vi "WellPartition_Index.vi"(2 "PartitionArray":string[](array[string])=["A, MQ unfiltered", "A, MQ unfiltered", "A, MQ unfiltered", "B, D2O unfiltered", "B, D2O unfiltered", "B, D2O unfiltered", "C, 1mg/ml Snomax in MQ", "C, 1mg/ml Snomax in MQ", "C, 1mg/ml Snomax in MQ", "C, 1mg/ml Snomax in MQ", "C, 1mg/ml Snomax in MQ", "C, 1mg/ml Snomax in MQ", "D, 1mg/ml Snomax in 1:1 MQ:D2O", "D, 1mg/ml Snomax in 1:1 MQ:D2O", "D, 1mg/ml Snomax in 1:1 MQ:D2O", "D, 1mg/ml Snomax in 1:1 MQ:D2O", "D, 1mg/ml Snomax in 1:1 MQ:D2O", "D, 1mg/ml Snomax in 1:1 MQ:D2O", "E, 1mg/ml Snomax in D2O", "E, 1mg/ml Snomax in D2O", "E, 1mg/ml Snomax in D2O", "E, 1mg/ml Snomax in D2O", "E, 1mg/ml Snomax in D2O", "E, 1mg/ml Snomax in D2O", "A, MQ unfiltered", "A, MQ unfiltered", "A, MQ unfiltered", "B, D2O unfiltered", "B, D2O unfiltered", "B, D2O unfiltered", "C, 1mg/ml Snomax in MQ", "C, 1mg/ml Snomax in MQ", "C, 1mg/ml Snomax in MQ", "C, 1mg/ml Snomax in MQ", "C, 1mg/ml Snomax in MQ", "C, 1mg/ml Snomax in MQ", "D, 1mg/ml Snomax in 1:1 MQ:D2O", "D, 1mg/ml Snomax in 1:1 MQ:D2O", "D, 1mg/ml Snomax in 1:1 MQ:D2O", "D, 1mg/ml Snomax in 1:1 MQ:D2O", "D, 1mg/ml Snomax in 1:1 MQ:D2O", "D, 1mg/ml Snomax in 1:1 MQ:D2O", "E, 1mg/ml Snomax in D2O", "E, 1mg/ml Snomax in D2O", "E, 1mg/ml Snomax in D2O", "E, 1mg/ml Snomax in D2O", "E, 1mg/ml Snomax in D2O", "E, 1mg/ml Snomax in D2O", "A, MQ unfiltered", "A, MQ unfiltered", "A, MQ unfiltered", "B, D2O unfiltered", "B, D2O unfiltered", "B, D2O unfiltered", "C, 1mg/ml Snomax in MQ", "C, 1mg/ml Snomax in MQ", "C, 1mg/ml Snomax in MQ", "C, 1mg/ml Snomax in MQ", "C, 1mg/ml Snomax in MQ", "C, 1mg/ml Snomax in MQ", "D, 1mg/ml Snomax in 1:1 MQ:D2O", "D, 1mg/ml Snomax in 1:1 MQ:D2O", "D, 1mg/ml Snomax in 1:1 MQ:D2O", "D, 1mg/ml Snomax in 1:1 MQ:D2O", "D, 1mg/ml Snomax in 1:1 MQ:D2O", "D, 1mg/ml Snomax in 1:1 MQ:D2O", "E, 1mg/ml Snomax in D2O", "E, 1mg/ml Snomax in D2O", "E, 1mg/ml Snomax in D2O", "E, 1mg/ml Snomax in D2O", "E, 1mg/ml Snomax in D2O", "E, 1mg/ml Snomax in D2O", "A, MQ unfiltered", "A, MQ unfiltered", "A, MQ unfiltered", "B, D2O unfiltered", "B, D2O unfiltered", "B, D2O unfiltered", "C, 1mg/ml Snomax in MQ", "C, 1mg/ml Snomax in MQ", "C, 1mg/ml Snomax in MQ", "C, 1mg/ml Snomax in MQ", "C, 1mg/ml Snomax in MQ", "C, 1mg/ml Snomax in MQ", "D, 1mg/ml Snomax in 1:1 MQ:D2O", "D, 1mg/ml Snomax in 1:1 MQ:D2O", "D, 1mg/ml Snomax in 1:1 MQ:D2O", "D, 1mg/ml Snomax in 1:1 MQ:D2O", "D, 1mg/ml Snomax in 1:1 MQ:D2O", "D, 1mg/ml Snomax in 1:1 MQ:D2O", "E, 1mg/ml Snomax in D2O", "E, 1mg/ml Snomax in D2O", "E, 1mg/ml Snomax in D2O", "E, 1mg/ml Snomax in D2O", "E, 1mg/ml Snomax in D2O", "E, 1mg/ml Snomax in D2O", "A, MQ unfiltered", "A, MQ unfiltered", "A, MQ unfiltered", "B, D2O unfiltered", "B, D2O unfiltered", "B, D2O unfiltered", "C, 1mg/ml Snomax in MQ", "C, 1mg/ml Snomax in MQ", "C, 1mg/ml Snomax in MQ", "C, 1mg/ml Snomax in MQ", "C, 1mg/ml Snomax in MQ", "C, 1mg/ml Snomax in MQ", "D, 1mg/ml Snomax in 1:1 MQ:D2O", "D, 1mg/ml Snomax in 1:1 MQ:D2O", "D, 1mg/ml Snomax in 1:1 MQ:D2O", "D, 1mg/ml Snomax in 1:1 MQ:D2O", "D, 1mg/ml Snomax in 1:1 MQ:D2O", "D, 1mg/ml Snomax in 1:1 MQ:D2O", "E, 1mg/ml Snomax in D2O", "E, 1mg/ml Snomax in D2O", "E, 1mg/ml Snomax in D2O", "E, 1mg/ml Snomax in D2O", "E, 1mg/ml Snomax in D2O", "E, 1mg/ml Snomax in D2O", "A, MQ unfiltered", "A, MQ unfiltered", "A, MQ unfiltered", "B, D2O unfiltered", "B, D2O unfiltered", "B, D2O unfiltered", "C, 1mg/ml Snomax in MQ", "C, 1mg/ml Snomax in MQ", "C, 1mg/ml Snomax in MQ", "C, 1mg/ml Snomax in MQ", "C, 1mg/ml Snomax in MQ", "C, 1mg/ml Snomax in MQ", "D, 1mg/ml Snomax in 1:1 MQ:D2O", "D, 1mg/ml Snomax in 1:1 MQ:D2O", "D, 1mg/ml Snomax in 1:1 MQ:D2O", "D, 1mg/ml Snomax in 1:1 MQ:D2O", "D, 1mg/ml Snomax in 1:1 MQ:D2O", "D, 1mg/ml Snomax in 1:1 MQ:D2O", "E, 1mg/ml Snomax in D2O", "E, 1mg/ml Snomax in D2O", "E, 1mg/ml Snomax in D2O", "E, 1mg/ml Snomax in D2O", "E, 1mg/ml Snomax in D2O", "E, 1mg/ml Snomax in D2O", "A, MQ unfiltered", "A, MQ unfiltered", "A, MQ unfiltered", "B, D2O unfiltered", "B, D2O unfiltered", "B, D2O unfiltered", "C, 1mg/ml Snomax in MQ", "C, 1mg/ml Snomax in MQ", "C, 1mg/ml Snomax in MQ", "C, 1mg/ml Snomax in MQ", "C, 1mg/ml Snomax in MQ", "C, 1mg/ml Snomax in MQ", "D, 1mg/ml Snomax in 1:1 MQ:D2O", "D, 1mg/ml Snomax in 1:1 MQ:D2O", "D, 1mg/ml Snomax in 1:1 MQ:D2O", "D, 1mg/ml Snomax in 1:1 MQ:D2O", "D, 1mg/ml Snomax in 1:1 MQ:D2O", "D, 1mg/ml Snomax in 1:1 MQ:D2O", "E, 1mg/ml Snomax in D2O", "E, 1mg/ml Snomax in D2O", "E, 1mg/ml Snomax in D2O", "E, 1mg/ml Snomax in D2O", "E, 1mg/ml Snomax in D2O", "E, 1mg/ml Snomax in D2O", "A, MQ unfiltered", "A, MQ unfiltered", "A, MQ unfiltered", "B, D2O unfiltered", "B, D2O unfiltered", "B, D2O unfiltered", "C, 1mg/ml Snomax in MQ", "C, 1mg/ml Snomax in MQ", "C, 1mg/ml Snomax in MQ", "C, 1mg/ml Snomax in MQ", "C, 1mg/ml Snomax in MQ", "C, 1mg/ml Snomax in MQ", "D, 1mg/ml Snomax in 1:1 MQ:D2O", "D, 1mg/ml Snomax in 1:1 MQ:D2O", "D, 1mg/ml Snomax in 1:1 MQ:D2O", "D, 1mg/ml Snomax in 1:1 MQ:D2O", "D, 1mg/ml Snomax in 1:1 MQ:D2O", "D, 1mg/ml Snomax in 1:1 MQ:D2O", "E, 1mg/ml Snomax in D2O", "E, 1mg/ml Snomax in D2O", "E, 1mg/ml Snomax in D2O", "E, 1mg/ml Snomax in D2O", "E, 1mg/ml Snomax in D2O", "E, 1mg/ml Snomax in D2O", "A, MQ unfiltered", "A, MQ unfiltered", "A, MQ unfiltered", "B, D2O unfiltered", "B, D2O unfiltered", "B, D2O unfiltered", "C, 1mg/ml Snomax in MQ", "C, 1mg/ml Snomax in MQ", "C, 1mg/ml Snomax in MQ", "C, 1mg/ml Snomax in MQ", "C, 1mg/ml Snomax in MQ", "C, 1mg/ml Snomax in MQ", "D, 1mg/ml Snomax in 1:1 MQ:D2O", "D, 1mg/ml Snomax in 1:1 MQ:D2O", "D, 1mg/ml Snomax in 1:1 MQ:D2O", "D, 1mg/ml Snomax in 1:1 MQ:D2O", "D, 1mg/ml Snomax in 1:1 MQ:D2O", "D, 1mg/ml Snomax in 1:1 MQ:D2O", "E, 1mg/ml Snomax in D2O", "E, 1mg/ml Snomax in D2O", "E, 1mg/ml Snomax in D2O", "E, 1mg/ml Snomax in D2O", "E, 1mg/ml Snomax in D2O", "E, 1mg/ml Snomax in D2O", "A, MQ unfiltered", "A, MQ unfiltered", "A, MQ unfiltered", "B, D2O unfiltered", "B, D2O unfiltered", "B, D2O unfiltered", "C, 1mg/ml Snomax in MQ", "C, 1mg/ml Snomax in MQ", "C, 1mg/ml Snomax in MQ", "C, 1mg/ml Snomax in MQ", "C, 1mg/ml Snomax in MQ", "C, 1mg/ml Snomax in MQ", "D, 1mg/ml Snomax in 1:1 MQ:D2O", "D, 1mg/ml Snomax in 1:1 MQ:D2O", "D, 1mg/ml Snomax in 1:1 MQ:D2O", "D, 1mg/ml Snomax in 1:1 MQ:D2O", "D, 1mg/ml Snomax in 1:1 MQ:D2O", "D, 1mg/ml Snomax in 1:1 MQ:D2O", "E, 1mg/ml Snomax in D2O", "E, 1mg/ml Snomax in D2O", "E, 1mg/ml Snomax in D2O", "E, 1mg/ml Snomax in D2O", "E, 1mg/ml Snomax in D2O", "E, 1mg/ml Snomax in D2O", "A, MQ unfiltered", "A, MQ unfiltered", "A, MQ unfiltered", "B, D2O unfiltered", "B, D2O unfiltered", "B, D2O unfiltered", "C, 1mg/ml Snomax in MQ", "C, 1mg/ml Snomax in MQ", "C, 1mg/ml Snomax in MQ", "C, 1mg/ml Snomax in MQ", "C, 1mg/ml Snomax in MQ", "C, 1mg/ml Snomax in MQ", "D, 1mg/ml Snomax in 1:1 MQ:D2O", "D, 1mg/ml Snomax in 1:1 MQ:D2O", "D, 1mg/ml Snomax in 1:1 MQ:D2O", "D, 1mg/ml Snomax in 1:1 MQ:D2O", "D, 1mg/ml Snomax in 1:1 MQ:D2O", "D, 1mg/ml Snomax in 1:1 MQ:D2O", "E, 1mg/ml Snomax in D2O", "E, 1mg/ml Snomax in D2O", "E, 1mg/ml Snomax in D2O", "E, 1mg/ml Snomax in D2O", "E, 1mg/ml Snomax in D2O", "E, 1mg/ml Snomax in D2O", "A, MQ unfiltered", "A, MQ unfiltered", "A, MQ unfiltered", "B, D2O unfiltered", "B, D2O unfiltered", "B, D2O unfiltered", "C, 1mg/ml Snomax in MQ", "C, 1mg/ml Snomax in MQ", "C, 1mg/ml Snomax in MQ", "C, 1mg/ml Snomax in MQ", "C, 1mg/ml Snomax in MQ", "C, 1mg/ml Snomax in MQ", "D, 1mg/ml Snomax in 1:1 MQ:D2O", "D, 1mg/ml Snomax in 1:1 MQ:D2O", "D, 1mg/ml Snomax in 1:1 MQ:D2O", "D, 1mg/ml Snomax in 1:1 MQ:D2O", "D, 1mg/ml Snomax in 1:1 MQ:D2O", "D, 1mg/ml Snomax in 1:1 MQ:D2O", "E, 1mg/ml Snomax in D2O", "E, 1mg/ml Snomax in D2O", "E, 1mg/ml Snomax in D2O", "E, 1mg/ml Snomax in D2O", "E, 1mg/ml Snomax in D2O", "E, 1mg/ml Snomax in D2O", "A, MQ unfiltered", "A, MQ unfiltered", "A, MQ unfiltered", "B, D2O unfiltered", "B, D2O unfiltered", "B, D2O unfiltered", "C, 1mg/ml Snomax in MQ", "C, 1mg/ml Snomax in MQ", "C, 1mg/ml Snomax in MQ", "C, 1mg/ml Snomax in MQ", "C, 1mg/ml Snomax in MQ", "C, 1mg/ml Snomax in MQ", "D, 1mg/ml Snomax in 1:1 MQ:D2O", "D, 1mg/ml Snomax in 1:1 MQ:D2O", "D, 1mg/ml Snomax in 1:1 MQ:D2O", "D, 1mg/ml Snomax in 1:1 MQ:D2O", "D, 1mg/ml Snomax in 1:1 MQ:D2O", "D, 1mg/ml Snomax in 1:1 MQ:D2O", "E, 1mg/ml Snomax in D2O", "E, 1mg/ml Snomax in D2O", "E, 1mg/ml Snomax in D2O", "E, 1mg/ml Snomax in D2O", "E, 1mg/ml Snomax in D2O", "E, 1mg/ml Snomax in D2O", "A, MQ unfiltered", "A, MQ unfiltered", "A, MQ unfiltered", "B, D2O unfiltered", "B, D2O unfiltered", "B, D2O unfiltered", "C, 1mg/ml Snomax in MQ", "C, 1mg/ml Snomax in MQ", "C, 1mg/ml Snomax in MQ", "C, 1mg/ml Snomax in MQ", "C, 1mg/ml Snomax in MQ", "C, 1mg/ml Snomax in MQ", "D, 1mg/ml Snomax in 1:1 MQ:D2O", "D, 1mg/ml Snomax in 1:1 MQ:D2O", "D, 1mg/ml Snomax in 1:1 MQ:D2O", "D, 1mg/ml Snomax in 1:1 MQ:D2O", "D, 1mg/ml Snomax in 1:1 MQ:D2O", "D, 1mg/ml Snomax in 1:1 MQ:D2O", "E, 1mg/ml Snomax in D2O", "E, 1mg/ml Snomax in D2O", "E, 1mg/ml Snomax in D2O", "E, 1mg/ml Snomax in D2O", "E, 1mg/ml Snomax in D2O", "E, 1mg/ml Snomax in D2O", "A, MQ unfiltered", "A, MQ unfiltered", "A, MQ unfiltered", "B, D2O unfiltered", "B, D2O unfiltered", "B, D2O unfiltered", "C, 1mg/ml Snomax in MQ", "C, 1mg/ml Snomax in MQ", "C, 1mg/ml Snomax in MQ", "C, 1mg/ml Snomax in MQ", "C, 1mg/ml Snomax in MQ", "C, 1mg/ml Snomax in MQ", "D, 1mg/ml Snomax in 1:1 MQ:D2O", "D, 1mg/ml Snomax in 1:1 MQ:D2O", "D, 1mg/ml Snomax in 1:1 MQ:D2O", "D, 1mg/ml Snomax in 1:1 MQ:D2O", "D, 1mg/ml Snomax in 1:1 MQ:D2O", "D, 1mg/ml Snomax in 1:1 MQ:D2O", "E, 1mg/ml Snomax in D2O", "E, 1mg/ml Snomax in D2O", "E, 1mg/ml Snomax in D2O", "E, 1mg/ml Snomax in D2O", "E, 1mg/ml Snomax in D2O", "E, 1mg/ml Snomax in D2O", "A, MQ unfiltered", "A, MQ unfiltered", "A, MQ unfiltered", "B, D2O unfiltered", "B, D2O unfiltered", "B, D2O unfiltered", "C, 1mg/ml Snomax in MQ", "C, 1mg/ml Snomax in MQ", "C, 1mg/ml Snomax in MQ", "C, 1mg/ml Snomax in MQ", "C, 1mg/ml Snomax in MQ", "C, 1mg/ml Snomax in MQ", "D, 1mg/ml Snomax in 1:1 MQ:D2O", "D, 1mg/ml Snomax in 1:1 MQ:D2O", "D, 1mg/ml Snomax in 1:1 MQ:D2O", "D, 1mg/ml Snomax in 1:1 MQ:D2O", "D, 1mg/ml Snomax in 1:1 MQ:D2O", "D, 1mg/ml Snomax in 1:1 MQ:D2O", "E, 1mg/ml Snomax in D2O", "E, 1mg/ml Snomax in D2O", "E, 1mg/ml Snomax in D2O", "E, 1mg/ml Snomax in D2O", "E, 1mg/ml Snomax in D2O", "E, 1mg/ml Snomax in D2O"], 3 "Well":i32=94) -> (0 "Unique Part Array":string[](array[string]), 1 "Partition Index":i32)   [LabVIEW 2022 SP3]
uses:
  6893864c-8b95-46b0-a9dc-c5db2e40fe38.vi
  6893864c-8b95-46b0-a9dc-c5db2e40fe38.vi/d4db2432-cc9c-482c-8957-dac855435ef6.vi
  6893864c-8b95-46b0-a9dc-c5db2e40fe38.vi/86fbf154-bd7b-49a2-8ab2-a837b2a95f24.vi
  6893864c-8b95-46b0-a9dc-c5db2e40fe38.vi/3b95b01e-1ec2-4565-bcd9-7606a5281010.vi
  6893864c-8b95-46b0-a9dc-c5db2e40fe38.vi/96a08935-737a-44b2-979c-a81d56408f7e.vi
  6893864c-8b95-46b0-a9dc-c5db2e40fe38.vi/d4db2432-cc9c-482c-8957-dac855435ef6.vi/6eaecd13-6e48-4772-a921-b51ebdf84d88.vi
  6893864c-8b95-46b0-a9dc-c5db2e40fe38.vi/d4db2432-cc9c-482c-8957-dac855435ef6.vi/d2d5f2b7-06f4-47f6-971c-049c3fdbb653.vi
  6893864c-8b95-46b0-a9dc-c5db2e40fe38.vi/3b95b01e-1ec2-4565-bcd9-7606a5281010.vi/6eaecd13-6e48-4772-a921-b51ebdf84d88.vi
  6893864c-8b95-46b0-a9dc-c5db2e40fe38.vi/3b95b01e-1ec2-4565-bcd9-7606a5281010.vi/d2d5f2b7-06f4-47f6-971c-049c3fdbb653.vi
  6893864c-8b95-46b0-a9dc-c5db2e40fe38.vi/96a08935-737a-44b2-979c-a81d56408f7e.vi/6eaecd13-6e48-4772-a921-b51ebdf84d88.vi
  6893864c-8b95-46b0-a9dc-c5db2e40fe38.vi/96a08935-737a-44b2-979c-a81d56408f7e.vi/d2d5f2b7-06f4-47f6-971c-049c3fdbb653.vi
  <vilib>/Comparison/Less/Less Functor/Less Functor.lvclass
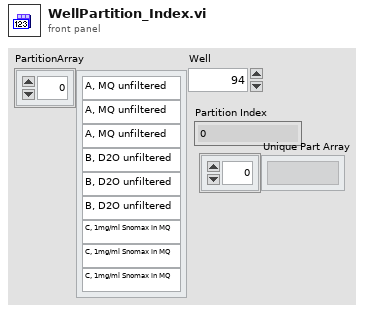
[diagram p1: front panel]
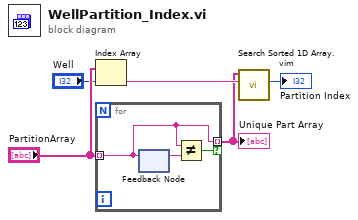
[diagram p0: block diagram]
diagram:
  n1 = Index Array(array="PartitionArray", index="Well") -> (element=w3:string)
  n2 = for {
    tunnel: "PartitionArray" -> [w7] mode=indexing
    tunnel: [w7] -> w2 mode=indexing if=w6
    n3 = feedback-in #1(w7) -> ()
    n4 = feedback #1() -> (w8:string)  [unwired: 1 in]
    n5 = Not Equal?(x=w7, y=w8) -> (x != y?=w6:bool)
  }
  "Unique Part Array" <- w2
  n6 = call "Search Sorted 1D Array.vim"("element"=w3, "sorted 1D array"=w2) -> ("nearest index"=→"Partition Index":i32)  [unwired: 8 in, 1 out]
